vi "Set Vel Accel Decel.vi"(8 "error in (no error)":errorcluster, 10 "Motion Parameters In":T2, 11 "Port In":T3) -> (0 "error out":errorcluster, 2 "Motion Parameters Out":T1, 3 "Port Out":T3)   [LabVIEW 2021]
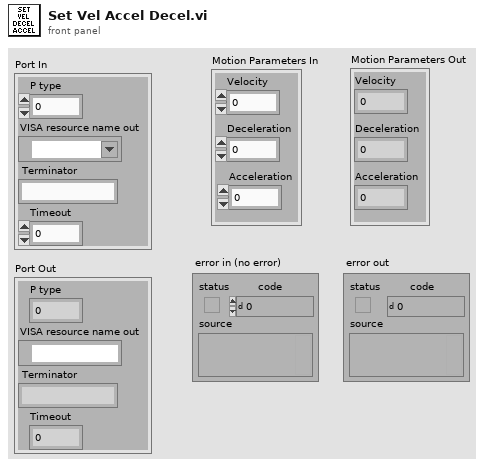
[diagram p1: front panel]
types:
  T1 = cluster{"Velocity ":dbl, "Deceleration ":dbl, "Acceleration":dbl}
  T2 = cluster{"Velocity":dbl, "Deceleration ":dbl, "Acceleration":dbl}
  T3 = cluster{"P type":u16, "VISA resource name out":refnum<visa-resource-name>, " Terminator":string, "Timeout":i32}
  T4 = cluster{"velocity out":dbl, "deceleration out":dbl, "accel out":dbl}
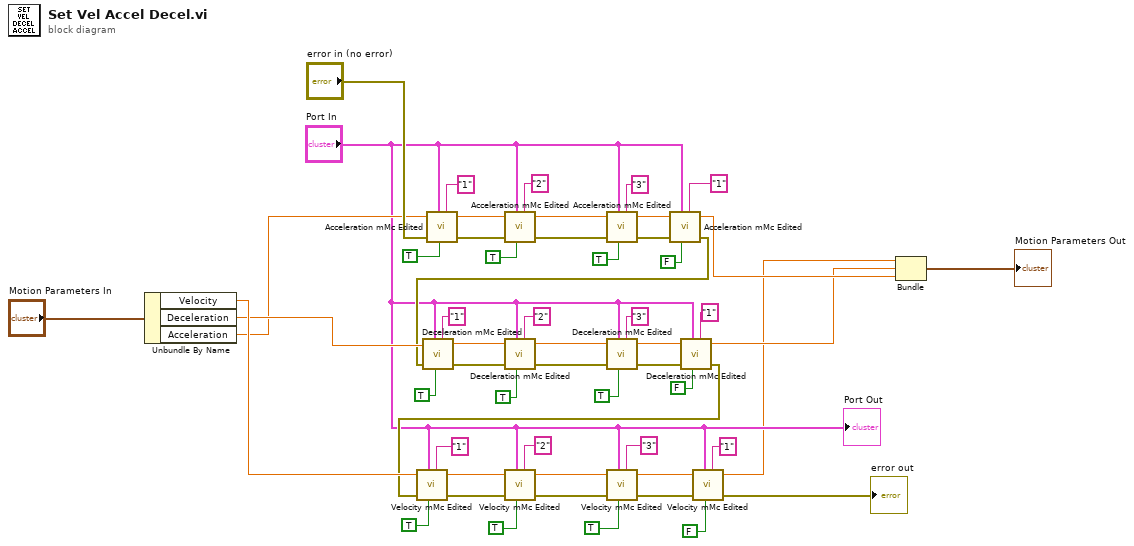
[diagram p0: block diagram]
diagram:
  n1 = Unbundle By Name("Motion Parameters In") -> ("Velocity"=w24:dbl, "Deceleration"=w23:dbl, "Acceleration"=w22:dbl)
  n2 = call "Acceleration mMc Edited.vi"("accel in"=w22, "Port"="Port In", "error in (no error)"="error in (no error)", "set/get"=TRUE, "Controller #"="1") -> ("accel out"=w51:dbl, "error out"=w49:errorcluster)  [unwired: 3 in]
  n3 = call "Acceleration mMc Edited.vi"("accel in"=w51, "Port"="Port In", "error in (no error)"=w49, "set/get"=TRUE, "Controller #"="2") -> ("accel out"=w50:dbl, "error out"=w48:errorcluster)  [unwired: 3 in]
  n4 = call "Acceleration mMc Edited.vi"("accel in"=w50, "Port"="Port In", "error in (no error)"=w48, "set/get"=TRUE, "Controller #"="3") -> ("accel out"=w18:dbl, "error out"=w14:errorcluster)  [unwired: 3 in]
  n5 = call "Acceleration mMc Edited.vi"("accel in"=w18, "Port"="Port In", "error in (no error)"=w14, "set/get"=FALSE, "Controller #"="1") -> ("accel out"=w17:dbl, "error out"=w15:errorcluster)  [unwired: 3 in]
  n6 = call "Deceleration mMc Edited.vi"("deceleration in"=w23, "Port"="Port In", "error in (no error)"=w15, "set/get"=TRUE, "Controller #"="1") -> ("deceleration out"=w53:dbl, "error out"=w47:errorcluster)  [unwired: 3 in]
  n7 = call "Deceleration mMc Edited.vi"("deceleration in"=w53, "Port"="Port In", "error in (no error)"=w47, "set/get"=TRUE, "Controller #"="2") -> ("deceleration out"=w52:dbl, "error out"=w46:errorcluster)  [unwired: 3 in]
  n8 = call "Deceleration mMc Edited.vi"("deceleration in"=w52, "Port"="Port In", "error in (no error)"=w46, "set/get"=TRUE, "Controller #"="3") -> ("deceleration out"=w13:dbl, "error out"=w10:errorcluster)  [unwired: 3 in]
  n9 = call "Deceleration mMc Edited.vi"("deceleration in"=w13, "Port"="Port In", "error in (no error)"=w10, "set/get"=FALSE, "Controller #"="1") -> ("deceleration out"=w12:dbl, "error out"=w9:errorcluster)  [unwired: 3 in]
  n10 = call "Velocity mMc Edited.vi"("velocity in"=w24, "Port"="Port In", "error in (no error)"=w9, "set/get"=TRUE, "Controller #"="1") -> ("velocity out"=w55:dbl, "error out"=w45:errorcluster)  [unwired: 3 in]
  n11 = call "Velocity mMc Edited.vi"("velocity in"=w55, "Port"="Port In", "error in (no error)"=w45, "set/get"=TRUE, "Controller #"="2") -> ("velocity out"=w54:dbl, "error out"=w44:errorcluster)  [unwired: 3 in]
  n12 = call "Velocity mMc Edited.vi"("velocity in"=w54, "Port"="Port In", "error in (no error)"=w44, "set/get"=TRUE, "Controller #"="3") -> ("velocity out"=w4:dbl, "error out"=w8:errorcluster)  [unwired: 3 in]
  n13 = call "Velocity mMc Edited.vi"("velocity in"=w4, "Port"="Port In", "error in (no error)"=w8, "set/get"=FALSE, "Controller #"="1") -> ("velocity out"=w3:dbl, "error out"=→"error out":errorcluster)  [unwired: 3 in]
  n14 = Bundle("velocity out"=w3, "deceleration out"=w12, "accel out"=w17) -> (→"Motion Parameters Out":T4)  [unwired: 1 in]
  "Port Out" <- "Port In"
